vi "test_pid_v2.vi"() -> ()   [LabVIEW 2016]
uses:
  <vilib>/rvi/DesktopExecutionNode/Execution/niFpgaDEN_Execute.vi
  <vilib>/rvi/DesktopExecutionNode/DesktopExecutionNode.xnode
panel:
  in  "feedbaclTurnOnOff":i32[](array[numeric])
  in  "manMotTurnOnOff":i32[](array[numeric])
  in  "inputInvertPoint":i32
  in  "doMoveTime":i32
  out "simulationProgess":dbl(slide) scale=0.0..1.0
  out "position":dbl[](graph)
  out "Array":T1(array[cluster])
  in  "simTicks":i32
  in  "manualMotion":T2
  in  "liftOffParams":T3
  in  "fbParams":T4
  in  "input":fxp<+/-,24,16> format="%#_13g"
  in  "limits":T5
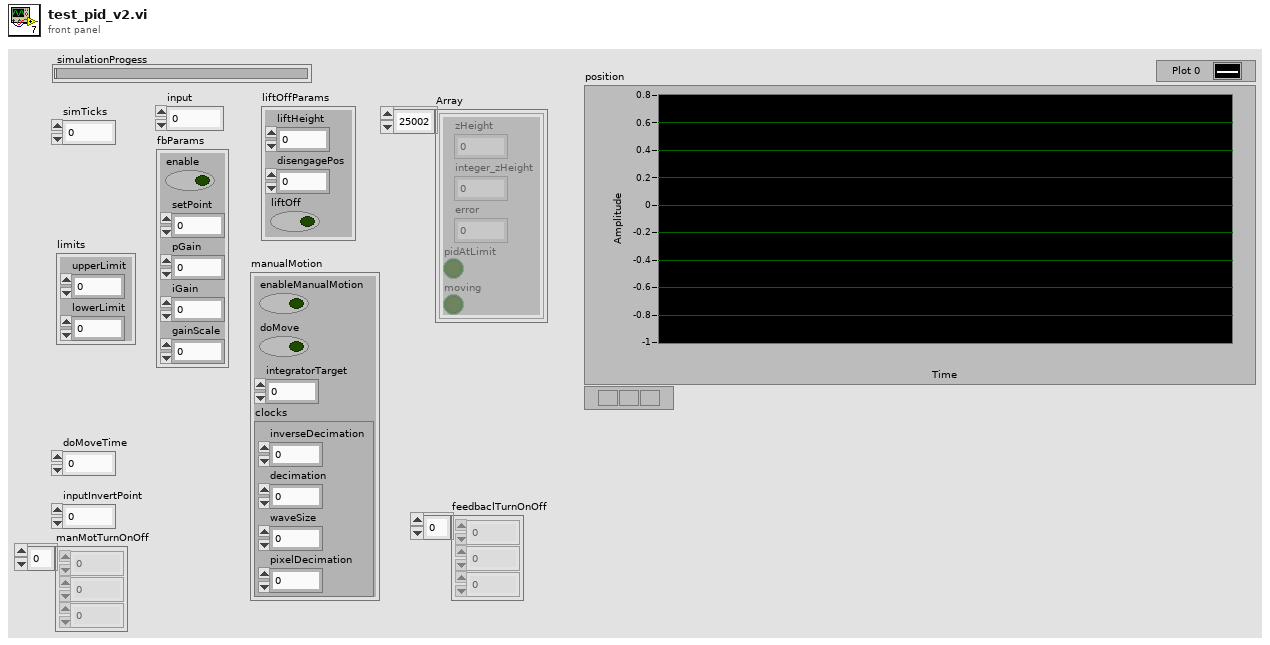
[diagram p1: front panel]
types:
  T1 = cluster{"zHeight":fxp<+/-,28,1>, "integer_zHeight":i16, "error":fxp<+/-,25,2>, "pidAtLimit":bool, "moving":bool}[]
  T2 = cluster{"enableManualMotion":bool, "doMove":bool, "integratorTarget":fxp<+/-,22,2>, "clocks":cluster{"inverseDecimation":fxp<+,22,0>, "decimation":u16, "waveSize":u16, "pixelDecimation":u16}}
  T3 = cluster{"liftHeight":fxp<+/-,15,4>, "disengagePos":fxp<+/-,22,1>, "liftOff":bool}
  T4 = cluster{"enable":bool, "setPoint":fxp<+/-,17,1>, "pGain":fxp<+/-,20,4>, "iGain":fxp<+/-,20,1>, "gainScale":i8}
  T5 = cluster{"upperLimit":fxp<+/-,28,4>, "lowerLimit":fxp<+/-,28,4>}
  T6 = cluster{"zHeight":fxp<+/-,28,1>, "integer_zHeight":i16, "error":fxp<+/-,25,2>, "pidAtLimit":bool, "moving":bool}
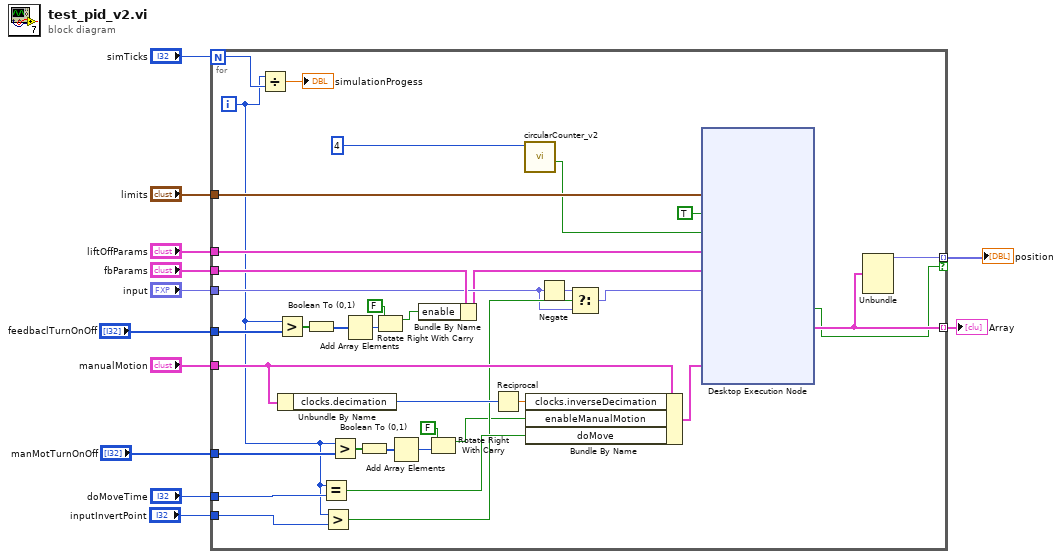
[diagram p0: block diagram]
diagram:
  n1 = for {
    N: "simTicks" -> [w36]
    tunnel: "limits" -> [w48]
    tunnel: [w44] -> w6 mode=indexing
    tunnel: "input" -> [w27]
    tunnel: "liftOffParams" -> [w46]
    tunnel: "fbParams" -> [w45]
    tunnel: "manualMotion" -> [w41]
    tunnel: [w43] -> w5 mode=indexing if=w42
    tunnel: "manMotTurnOnOff" -> [w34]
    tunnel: "doMoveTime" -> [w33]
    tunnel: "inputInvertPoint" -> [w30]
    tunnel: "feedbaclTurnOnOff" -> [w15]
    i -> [w14]
    n2 = Divide(x=w14, y=w36) -> (x/y=→"simulationProgess":dbl)
    n3 = Greater?(x=w14, y=w15) -> (0:w16:bool[])
    n4 = Unbundle By Name(w41) -> ("clocks.decimation"=w40:u16)
    n5 = Boolean To (0,1)(Boolean=w16) -> (0, 1=w17:i16[])
    n6 = Equal?(x=w14, y=w33) -> (x = y?=w32:bool)
    n7 = Greater?(x=w14, y=w30) -> (0:w28:bool)
    n8 = Greater?(x=w14, y=w34) -> (0:w25:bool[])
    n9 = Add Array Elements(numeric array=w17) -> (sum=w18:i16)
    n10 = Boolean To (0,1)(Boolean=w25) -> (0, 1=w24:i16[])
    n11 = Rotate Right With Carry(2:w18, 3:FALSE ("carry")) -> (1:w13:bool)  [unwired: 1 out]
    n12 = Add Array Elements(numeric array=w24) -> (sum=w23:i16)
    n13 = Bundle By Name(cluster=w45, "enable"=w13) -> (w20:T4)
    n14 = Rotate Right With Carry(2:w23, 3:FALSE ("carry")) -> (1:w21:bool)  [unwired: 1 out]
    n15 = Reciprocal(x=w40) -> (1/x=w39:dbl)
    n16 = call "circularCounter_v2.vi"("maxCount"=u16 4) -> ("maxPulse"=w37:bool)  [unwired: 7 in, 3 out]
    n17 = Bundle By Name(cluster=w41, "clocks.inverseDecimation"=w39, "enableManualMotion"=w21, "doMove"=w32) -> (w31:T2)
    n18 = Negate(x=w27) -> (-x=w26:fxp<+/-,25,17>)
    n19 = Select(t=w26, s=w28, f=w27) -> (s? t:f=w29:fxp<+/-,25,17>)
    n20 = xnode "Desktop Execution Node"("limits"=w48, "ready for output (T)"=TRUE, "inputValid"=w37, "liftOffParams"=w46, "fbParams"=w20, "input"=w29, "manualMotion"=w31) -> ("output valid"=w42:bool, "output"=w44:T6)  [unwired: 1 in, 2 out]
    n21 = Unbundle(w44) -> ("zHeight"=w43:fxp<+/-,28,1>)  [unwired: 4 out]
  }
  "Array" <- w6
  "position" <- w5
